vi "BL_UpdateParameters.vi"(0 "Potentiostat Galvanostat in":refnum<class "Potentiostat Galvanostat.lvclass">, 1 "Channel":u8 max=15, 2 "Techique Index":i32, 3 "Technique File Name (.ecc)":string, 4 "Technique Parameters":T1 {"Parameter Type" items=["I32 (Long)", "BOOL (Boolean)", "SGL (Single Precision)"]}, 5 "error in (no error)":errorcluster) -> (14 "Potentiostat Galvanostat out":refnum<class "Potentiostat Galvanostat.lvclass">, 15 "Channel":u8, 19 "error out":errorcluster)   [LabVIEW 2018, in "Potentiostat Galvanostat.lvclass"]
doc: "This function tests the communication speed between the library and the selected channel. \nNOTE: This function is for advanced user only."
uses:
  Potentiostat Galvanostat.lvclass
  Controls/Technique Parameters.ctl
  Controls/Technique Parameter.ctl
  Controls/Parameter Type.ctl
  Potentiostat Galvanostat.lvclass/Potentiostat Galvanostat.ctl
  BL_GetErrorMsg.vi
  <vilib>/Utility/error.llb/Error Cluster From Error Code.vi
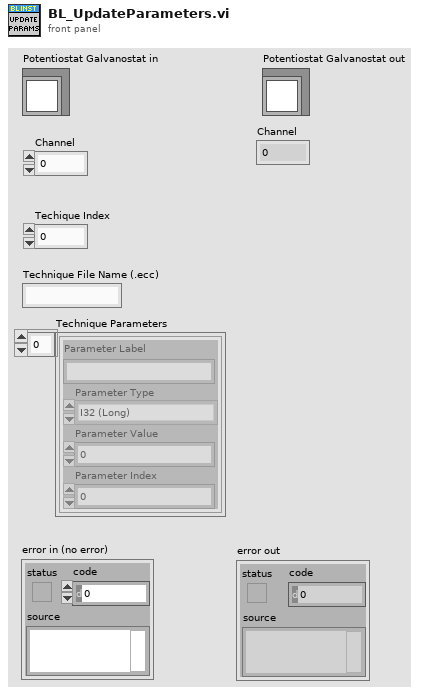
[diagram p1: front panel]
types:
  T1 = typedef "Potentiostat Galvanostat.lvclass/Technique Parameters.ctl" = T2[]
  T2 = typedef "Potentiostat Galvanostat.lvclass/Technique Parameter.ctl" = cluster{"Parameter Label":string, "Parameter Type":T3, "Parameter Value":i32, "Parameter Index":i32}
  T3 = typedef "Potentiostat Galvanostat.lvclass/Parameter Type.ctl" = i32
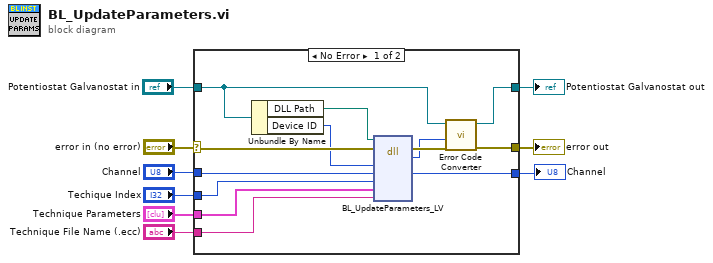
[diagram p0: block diagram]
diagram:
  n1 = case shown="No Error" "error in (no error)" {
    selector: "error in (no error)" -> [w18 w24]
    tunnel: [w22 w24] -> w8
    tunnel: [w20 w23] -> w6
    tunnel: "Potentiostat Galvanostat in" -> [w21 w23]
    tunnel: "Channel" -> [w15 _]
    tunnel: "Technique File Name (.ecc)" -> [w10 _]
    tunnel: "Technique Parameters" -> [w11 _]
    tunnel: [w14 _] -> w2
    tunnel: "Techique Index" -> [w12 _]
    frame No Error {
      n2 = Unbundle By Name(w21) -> ("DLL Path"=w16:path, "Device ID"=w17:i32)
      n3 = dll-call lib="C:/Projects/LabVIEW/BioLogic Instrument Driver/libs/EC-Lab Development Package/EClib.dll" fn="BL_UpdateParameters_LV"(path in=w16, error in=w18, "Device ID"=w17, "Channel"=w15, "Techique Index"=w12, "Technique Parameters"=w11, "Technique File Name(.ecc)"=w10) -> (error out=w19:errorcluster, "Error Code"=w13:i32, "Channel"=w14:u8)  [unwired: 5 in, 1 out]
      n4 = call "Error Code Converter.vi"("error in (no error)"=w19, "Error Code"=w13, "Potentiostat Galvanostat in"=w21) -> ("error out"=w22:errorcluster, "Potentiostat Galvanostat out"=w20:refnum<class "Potentiostat Galvanostat.lvclass">)  [unwired: 7 in]
    }
    frame Error {
    }
  }
  "error out" <- w8
  "Potentiostat Galvanostat out" <- w6
  "Channel" <- w2
